vi "Read String.vi"(11 "String With Equals in":refnum<class "String Without Equals.lvclass">) -> (2 "string":string, 3 "String With Equals out":refnum<class "String Without Equals.lvclass">)   [LabVIEW 2023, in "String Without Equals.lvclass"]
uses:
  String Without Equals.lvclass
  String Without Equals.lvclass/String Without Equals.ctl
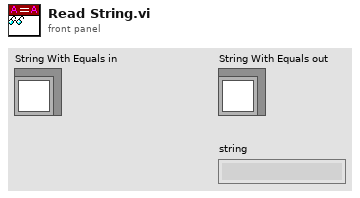
[diagram p1: front panel]
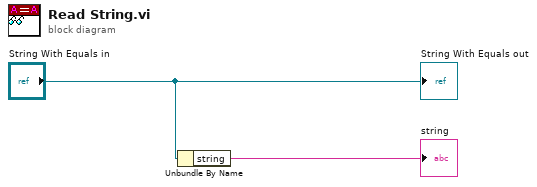
[diagram p0: block diagram]
diagram:
  n1 = Unbundle By Name("String With Equals in") -> ("string"=→"string":string)
  "String With Equals out" <- "String With Equals in"
